vi "0 Main Application - Energy Usage Version B.vi"() -> ()   [LabVIEW 2018]
panel:
  out "selected file path":path
  out "Min Cluster":T1 {"Hour" format="%<%H:%M>t"}
  out "Max cluster":T2 {"Hour" format="%<%H:%M>t"}
  out "results  data file path":path
  in  "Print Button":bool
  out "Total usage per day (KWh)":dbl
  out "Total (kWh/day)":dbl[](array[numeric])
  in  "Just Week days":bool
  out "G-6:15PM-8:00PM":dbl format="%.1f"
  out "H-8:15PM-10:00PM":dbl format="%.1f"
  out "F-4:15PM-6:00PM":dbl format="%.1f"
  out "E-2:15PM-4:00PM":dbl format="%.1f"
  out "D-12:15 -2:00PM":dbl format="%.1f"
  out "C-10:15-12:00":dbl format="%.1f"
  out "B-8:15-10:00":dbl format="%.1f"
  out "A-6:15-8:00":dbl format="%.1f"
  out "Average usage":dbl[][](graph)
  out "standard deviation":dbl format="%0.2f"
  out "actual data":dbl[][](array[numeric])
  in  "Remove weekday fltr":bool
  in  "Weekday filter":T3
  in  "Remove filter":bool
  in  "Quarter Filter":T4 {"month ring" items=["Jan", "Feb", "Mar", "Apr", "May", "Jun", "Jul", "Ago", "Set", "Oct", "Nov", "Dec"]}
  in  "Tab Control":enum32{"per hour", "Total /day"}(tab)
  out "Per Hour":cluster{"Y":dbl[], "Y":dbl[]}[](graph)
  out "Average Demand (kW)":dbl format="%#.2g"
  out "Total Demand (KWh)":dbl format="%.2f"
  out "Total per day":cluster{"Y":dbl[], "Y":dbl[]}[](graph)
  out "Average Demand (KWh/day)":dbl
  in  "SAVE PEAK DATA":bool
  out "%":dbl[](array[numeric]) format="%.2f"
  out "Demand (KW)":dbl
  out "Profile per day":dbl[][](graph)
  out "Peaks":cluster{i32[], dbl[]}[](graph)
  out "Hour":i32 format="%<%H:%M>t"
  out "Energy Usage":dbl[][](graph)
  in  "Read file":bool
  in  "stop":bool
  out "Date":u16(ring) items=["Fri Jan 1 2010", "Sat Jan 2 2010", "Sun Jan 3 2010", "Mon Jan 4 2010", "Tue Jan 5 2010", "Wed Jan 6 2010", "Thu Jan 7 2010", "Fri Jan 8 2010", "Sat Jan 9 2010", "Sun Jan 10 2010", "Mon Jan 11 2010", "Tue Jan 12 2010", "Wed Jan 13 2010", "Thu Jan 14 2010", "Fri Jan 15 2010", "Sat Jan 16 2010", "Sun Jan 17 2010", "Mon Jan 18 2010", "Tue Jan 19 2010", "Wed Jan 20 2010", "Thu Jan 21 2010", "Fri Jan 22 2010", "Sat Jan 23 2010", "Sun Jan 24 2010", "Mon Jan 25 2010", "Tue Jan 26 2010", "Wed Jan 27 2010", "Thu Jan 28 2010", "Fri Jan 29 2010", "Sat Jan 30 2010", "Sun Jan 31 2010", "Mon Feb 1 2010", "Tue Feb 2 2010", "Wed Feb 3 2010", "Thu Feb 4 2010", "Fri Feb 5 2010", "Sat Feb 6 2010", "Sun Feb 7 2010", "Mon Feb 8 2010", "Tue Feb 9 2010", "Wed Feb 10 2010", "Thu Feb 11 2010", "Fri Feb 12 2010", "Sat Feb 13 2010", "Sun Feb 14 2010", "Mon Feb 15 2010", "Tue Feb 16 2010", "Wed Feb 17 2010", "Thu Feb 18 2010", "Fri Feb 19 2010", "Sat Feb 20 2010", "Sun Feb 21 2010", "Mon Feb 22 2010", "Tue Feb 23 2010", "Wed Feb 24 2010", "Thu Feb 25 2010", "Fri Feb 26 2010", "Sat Feb 27 2010", "Sun Feb 28 2010", "Mon Mar 1 2010", "Tue Mar 2 2010", "Wed Mar 3 2010", "Thu Mar 4 2010", "Fri Mar 5 2010", "Sat Mar 6 2010", "Sun Mar 7 2010", "Mon Mar 8 2010", "Tue Mar 9 2010", "Wed Mar 10 2010", "Thu Mar 11 2010", "Fri Mar 12 2010", "Sat Mar 13 2010", "Sun Mar 14 2010", "Mon Mar 15 2010", "Tue Mar 16 2010", "Wed Mar 17 2010", "Thu Mar 18 2010", "Fri Mar 19 2010", "Sat Mar 20 2010", "Sun Mar 21 2010", "Mon Mar 22 2010", "Tue Mar 23 2010", "Wed Mar 24 2010", "Thu Mar 25 2010", "Fri Mar 26 2010", "Sat Mar 27 2010", "Sun Mar 28 2010", "Mon Mar 29 2010", "Tue Mar 30 2010", "Wed Mar 31 2010", "Thu Apr 1 2010", "Fri Apr 2 2010", "Sat Apr 3 2010", "Sun Apr 4 2010", "Mon Apr 5 2010", "Tue Apr 6 2010", "Wed Apr 7 2010", "Thu Apr 8 2010", "Fri Apr 9 2010", "Sat Apr 10 2010", "Sun Apr 11 2010", "Mon Apr 12 2010", "Tue Apr 13 2010", "Wed Apr 14 2010", "Thu Apr 15 2010", "Fri Apr 16 2010", "Sat Apr 17 2010", "Sun Apr 18 2010", "Mon Apr 19 2010", "Tue Apr 20 2010", "Wed Apr 21 2010", "Thu Apr 22 2010", "Fri Apr 23 2010", "Sat Apr 24 2010", "Sun Apr 25 2010", "Mon Apr 26 2010", "Tue Apr 27 2010", "Wed Apr 28 2010", "Thu Apr 29 2010", "Fri Apr 30 2010", "Sat May 1 2010", "Sun May 2 2010", "Mon May 3 2010", "Tue May 4 2010", "Wed May 5 2010", "Thu May 6 2010", "Fri May 7 2010", "Sat May 8 2010", "Sun May 9 2010", "Mon May 10 2010", "Tue May 11 2010", "Wed May 12 2010", "Thu May 13 2010", "Fri May 14 2010", "Sat May 15 2010", "Sun May 16 2010", "Mon May 17 2010", "Tue May 18 2010", "Wed May 19 2010", "Thu May 20 2010", "Fri May 21 2010", "Sat May 22 2010", "Sun May 23 2010", "Mon May 24 2010", "Tue May 25 2010", "Wed May 26 2010", "Thu May 27 2010", "Fri May 28 2010", "Sat May 29 2010", "Sun May 30 2010", "Mon May 31 2010", "Tue Jun 1 2010", "Wed Jun 2 2010", "Thu Jun 3 2010", "Fri Jun 4 2010", "Sat Jun 5 2010", "Sun Jun 6 2010", "Mon Jun 7 2010", "Tue Jun 8 2010", "Wed Jun 9 2010", "Thu Jun 10 2010", "Fri Jun 11 2010", "Sat Jun 12 2010", "Sun Jun 13 2010", "Mon Jun 14 2010", "Tue Jun 15 2010", "Wed Jun 16 2010", "Thu Jun 17 2010", "Fri Jun 18 2010", "Sat Jun 19 2010", "Sun Jun 20 2010", "Mon Jun 21 2010", "Tue Jun 22 2010", "Wed Jun 23 2010", "Thu Jun 24 2010", "Fri Jun 25 2010", "Sat Jun 26 2010", "Sun Jun 27 2010", "Mon Jun 28 2010", "Tue Jun 29 2010", "Wed Jun 30 2010", "Thu Jul 1 2010", "Fri Jul 2 2010", "Sat Jul 3 2010", "Sun Jul 4 2010", "Mon Jul 5 2010", "Tue Jul 6 2010", "Wed Jul 7 2010", "Thu Jul 8 2010", "Fri Jul 9 2010", "Sat Jul 10 2010", "Sun Jul 11 2010", "Mon Jul 12 2010", "Tue Jul 13 2010", "Wed Jul 14 2010", "Thu Jul 15 2010", "Fri Jul 16 2010", "Sat Jul 17 2010", "Sun Jul 18 2010", "Mon Jul 19 2010", "Tue Jul 20 2010", "Wed Jul 21 2010", "Thu Jul 22 2010", "Fri Jul 23 2010", "Sat Jul 24 2010", "Sun Jul 25 2010", "Mon Jul 26 2010", "Tue Jul 27 2010", "Wed Jul 28 2010", "Thu Jul 29 2010", "Fri Jul 30 2010", "Sat Jul 31 2010", "Sun Aug 1 2010", "Mon Aug 2 2010", "Tue Aug 3 2010", "Wed Aug 4 2010", "Thu Aug 5 2010", "Fri Aug 6 2010", "Sat Aug 7 2010", "Sun Aug 8 2010", "Mon Aug 9 2010", "Tue Aug 10 2010", "Wed Aug 11 2010", "Thu Aug 12 2010", "Fri Aug 13 2010", "Sat Aug 14 2010", "Sun Aug 15 2010", "Mon Aug 16 2010", "Tue Aug 17 2010", "Wed Aug 18 2010", "Thu Aug 19 2010", "Fri Aug 20 2010", "Sat Aug 21 2010", "Sun Aug 22 2010", "Mon Aug 23 2010", "Tue Aug 24 2010", "Wed Aug 25 2010", "Thu Aug 26 2010", "Fri Aug 27 2010", "Sat Aug 28 2010", "Sun Aug 29 2010", "Mon Aug 30 2010", "Tue Aug 31 2010", "Wed Sep 1 2010", "Thu Sep 2 2010", "Fri Sep 3 2010", "Sat Sep 4 2010", "Sun Sep 5 2010", "Mon Sep 6 2010", "Tue Sep 7 2010", "Wed Sep 8 2010", "Thu Sep 9 2010", "Fri Sep 10 2010", "Sat Sep 11 2010", "Sun Sep 12 2010", "Mon Sep 13 2010", "Tue Sep 14 2010", "Wed Sep 15 2010", "Thu Sep 16 2010", "Fri Sep 17 2010", "Sat Sep 18 2010", "Sun Sep 19 2010", "Mon Sep 20 2010", "Tue Sep 21 2010", "Wed Sep 22 2010", "Thu Sep 23 2010", "Fri Sep 24 2010", "Sat Sep 25 2010", "Sun Sep 26 2010", "Mon Sep 27 2010", "Tue Sep 28 2010", "Wed Sep 29 2010", "Thu Sep 30 2010", "Fri Oct 1 2010", "Sat Oct 2 2010", "Sun Oct 3 2010", "Mon Oct 4 2010", "Tue Oct 5 2010", "Wed Oct 6 2010", "Thu Oct 7 2010", "Fri Oct 8 2010", "Sat Oct 9 2010", "Sun Oct 10 2010", "Mon Oct 11 2010", "Tue Oct 12 2010", "Wed Oct 13 2010", "Thu Oct 14 2010", "Fri Oct 15 2010", "Sat Oct 16 2010", "Sun Oct 17 2010", "Mon Oct 18 2010", "Tue Oct 19 2010", "Wed Oct 20 2010", "Thu Oct 21 2010", "Fri Oct 22 2010", "Sat Oct 23 2010", "Sun Oct 24 2010", "Mon Oct 25 2010", "Tue Oct 26 2010", "Wed Oct 27 2010", "Thu Oct 28 2010", "Fri Oct 29 2010", "Sat Oct 30 2010", "Sun Oct 31 2010", "Mon Nov 1 2010", "Tue Nov 2 2010", "Wed Nov 3 2010", "Thu Nov 4 2010", "Fri Nov 5 2010", "Sat Nov 6 2010", "Sun Nov 7 2010", "Mon Nov 8 2010", "Tue Nov 9 2010", "Wed Nov 10 2010", "Thu Nov 11 2010", "Fri Nov 12 2010", "Sat Nov 13 2010", "Sun Nov 14 2010", "Mon Nov 15 2010", "Tue Nov 16 2010", "Wed Nov 17 2010", "Thu Nov 18 2010", "Fri Nov 19 2010", "Sat Nov 20 2010", "Sun Nov 21 2010", "Mon Nov 22 2010", "Tue Nov 23 2010", "Wed Nov 24 2010", "Thu Nov 25 2010", "Fri Nov 26 2010", "Sat Nov 27 2010", "Sun Nov 28 2010", "Mon Nov 29 2010", "Tue Nov 30 2010", "Wed Dec 1 2010", "Thu Dec 2 2010", "Fri Dec 3 2010", "Sat Dec 4 2010", "Sun Dec 5 2010", "Mon Dec 6 2010", "Tue Dec 7 2010", "Wed Dec 8 2010", "Thu Dec 9 2010", "Fri Dec 10 2010", "Sat Dec 11 2010", "Sun Dec 12 2010", "Mon Dec 13 2010", "Tue Dec 14 2010", "Wed Dec 15 2010", "Thu Dec 16 2010", "Fri Dec 17 2010", "Sat Dec 18 2010", "Sun Dec 19 2010", "Mon Dec 20 2010", "Tue Dec 21 2010", "Wed Dec 22 2010", "Thu Dec 23 2010", "Fri Dec 24 2010", "Sat Dec 25 2010", "Sun Dec 26 2010", "Mon Dec 27 2010", "Tue Dec 28 2010", "Wed Dec 29 2010", "Thu Dec 30 2010", "Fri Dec 31 2010"]
  out "Peaks":dbl[](graph)
  # "A"
  # "B"
  # "C"
  # "D"
  # "E"
  # "F"
  # "G"
  # "H"
  # "```"
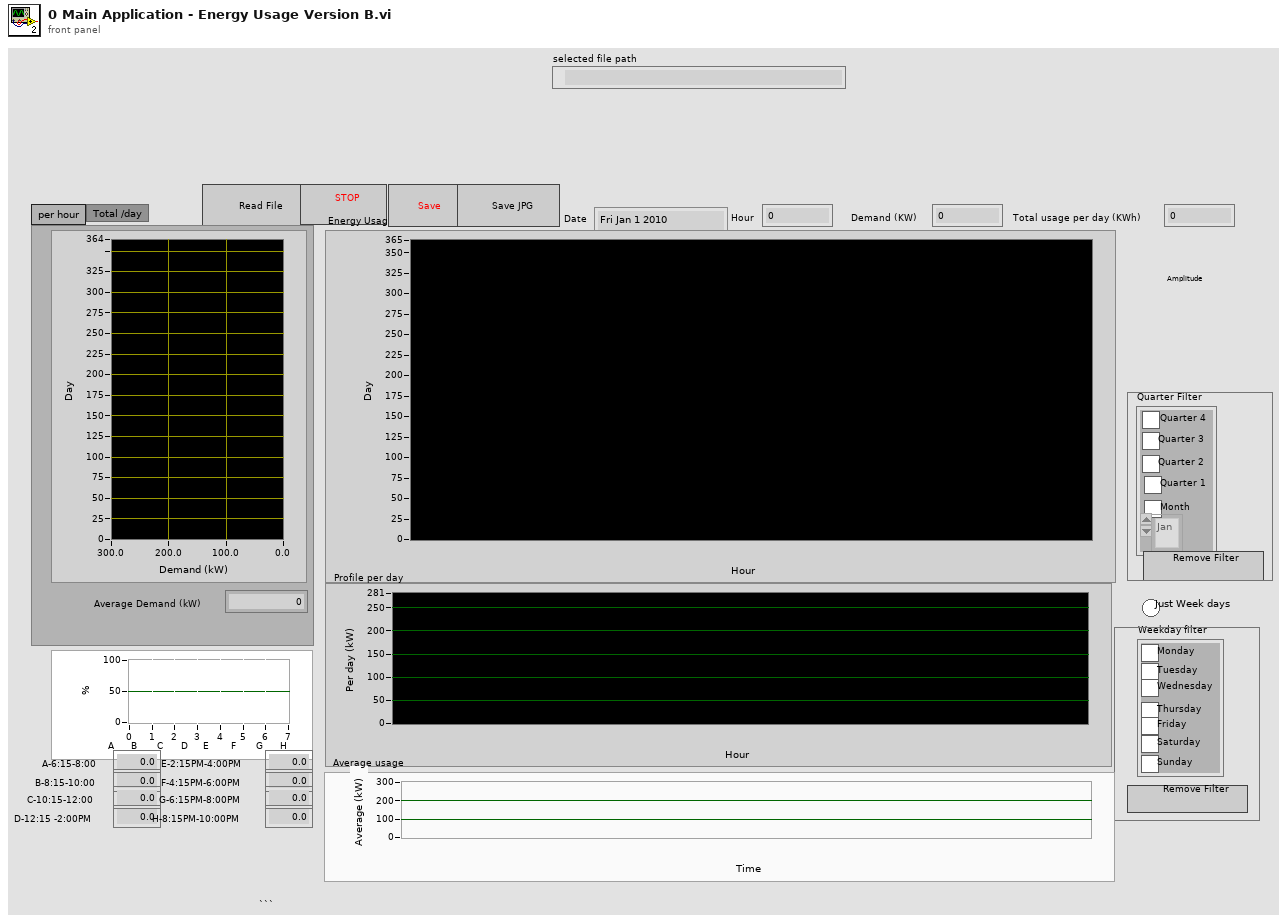
[diagram p1: front panel]
types:
  T1 = cluster{"Hour":i32, "min":dbl, "day of min":string}
  T2 = cluster{"Hour":i32, "Max peak":dbl, "day of max":string}
  T3 = cluster{"Monday":bool, "Tuesday":bool, "Wednesday":bool, "Thursday":bool, "Friday":bool, "Saturday":bool, "Sunday":bool}
  T4 = cluster{"Q1 3":bool, "Q2 2":bool, "Q3 2":bool, "Q4 2":bool, "Q1 4":bool, "month ring":u16}
  T5 = enum8{"Enabled", "Disabled", "Disabled and Grayed Out"}
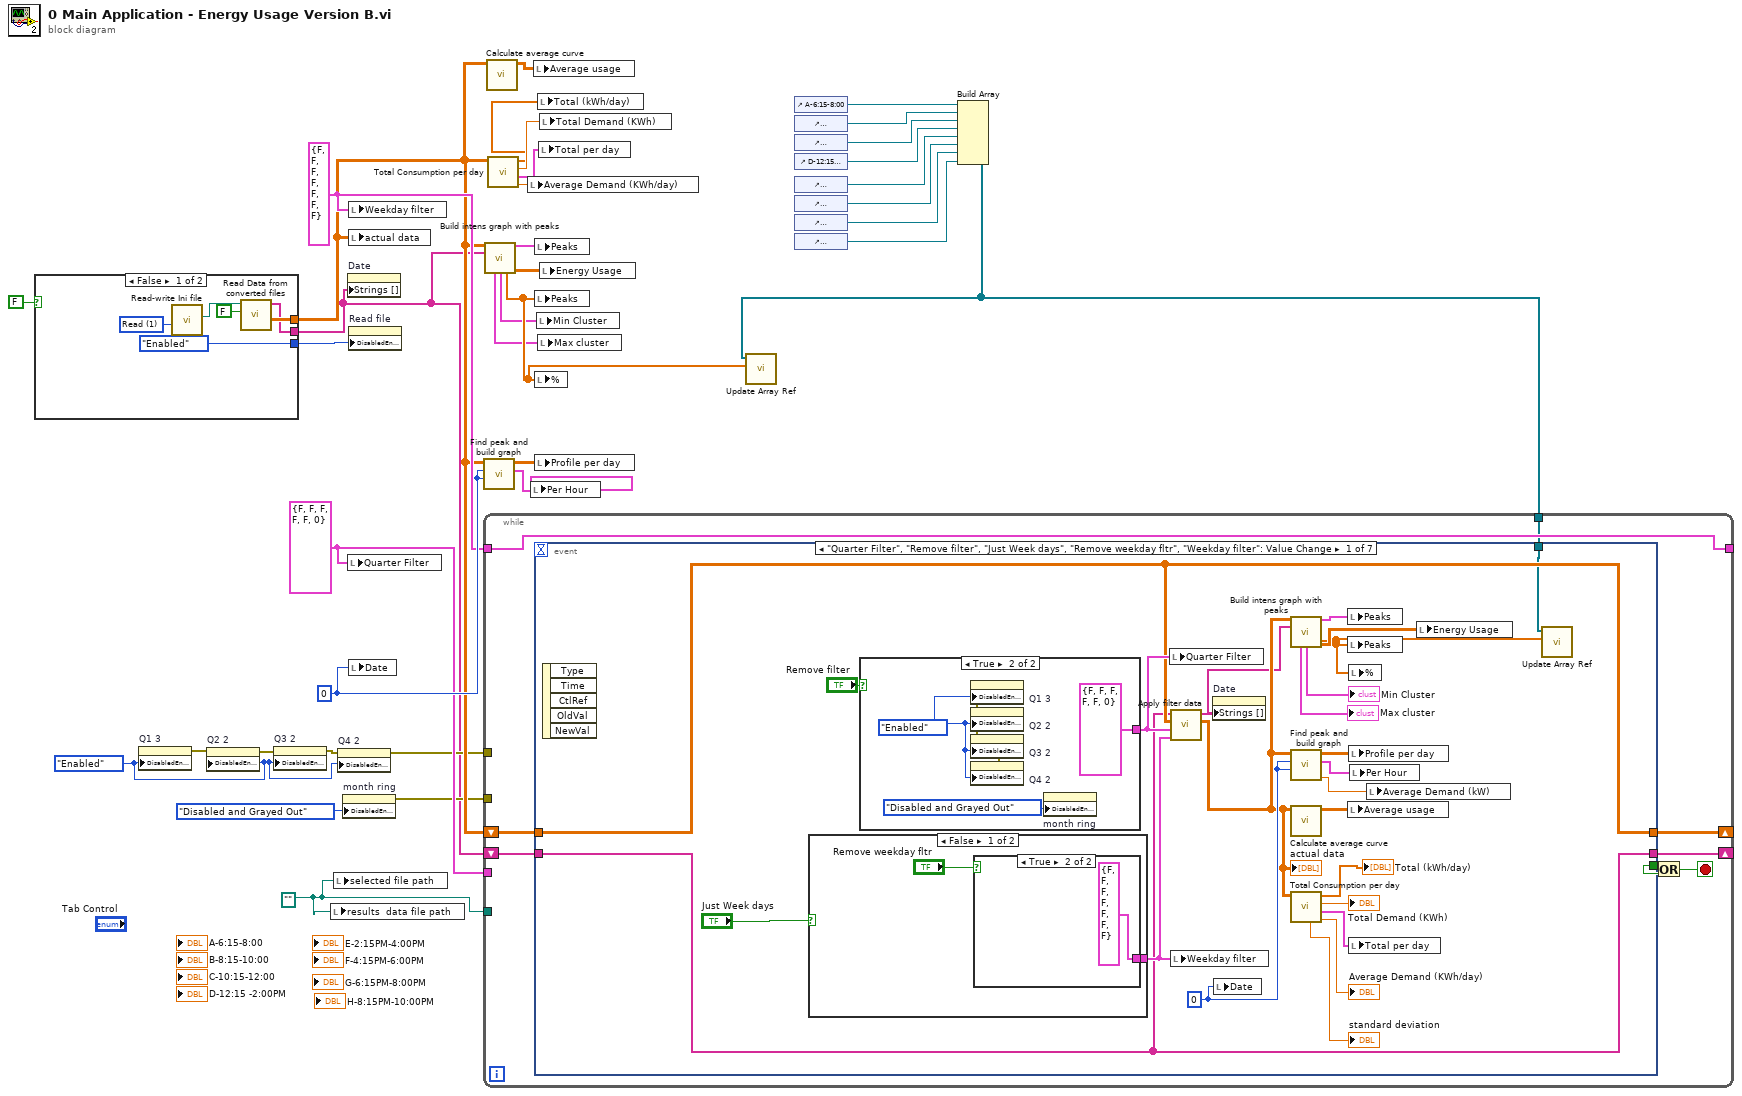
[diagram p0: block diagram]
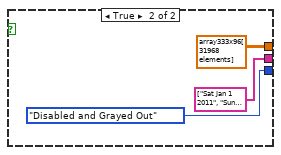
[diagram p2: hidden frame]
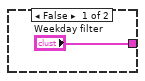
[diagram p3: hidden frame]
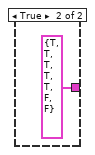
[diagram p4: hidden frame]
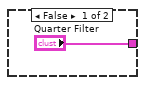
[diagram p5: hidden frame]
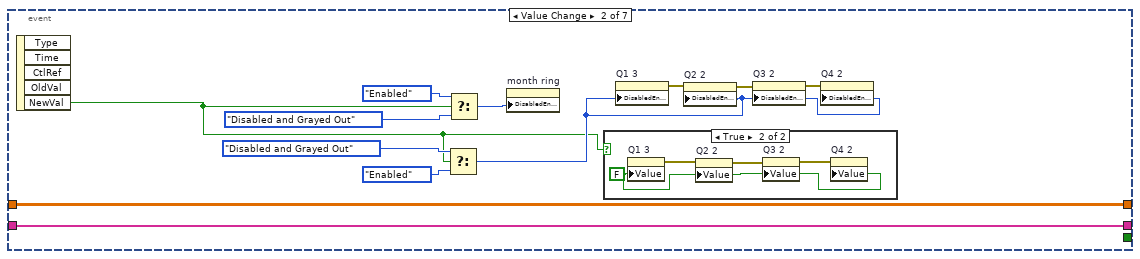
[diagram p6: hidden frame]
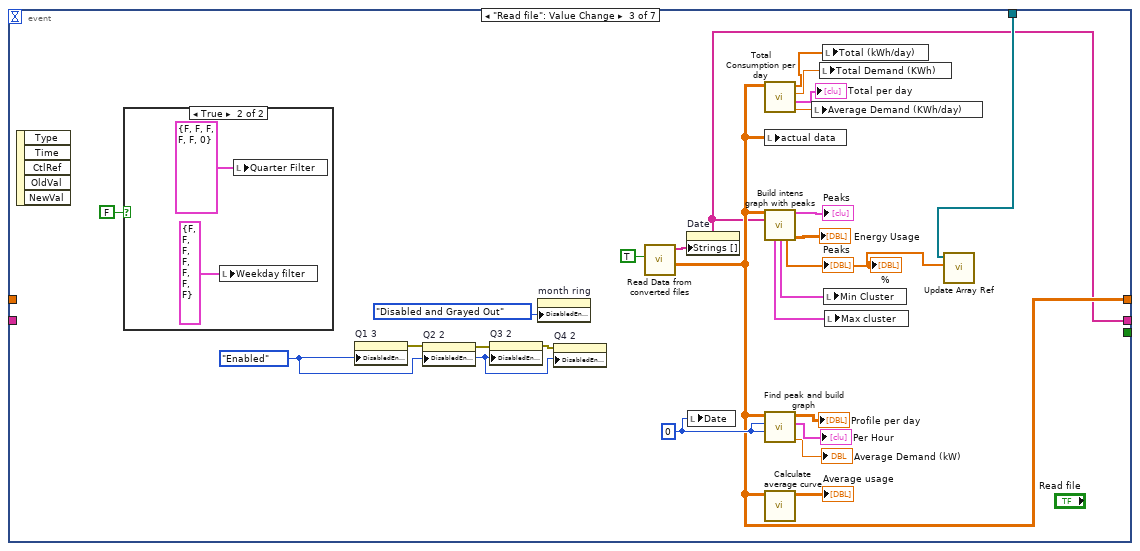
[diagram p8: hidden frame]
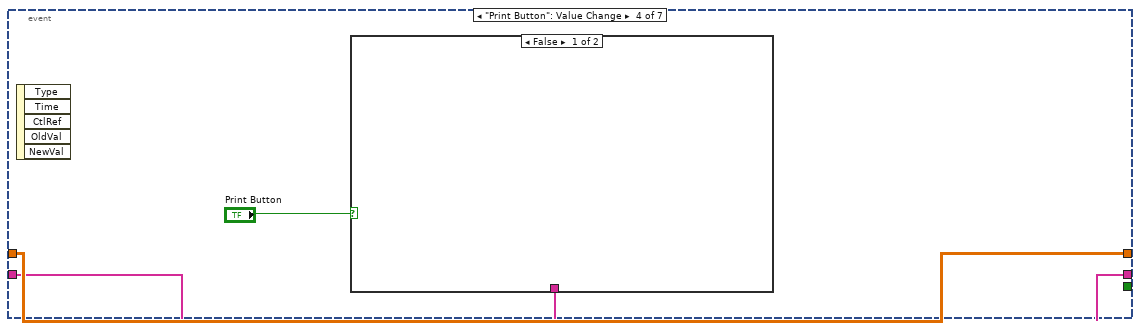
[diagram p10: hidden frame]
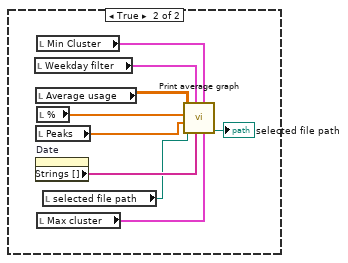
[diagram p11: hidden frame]
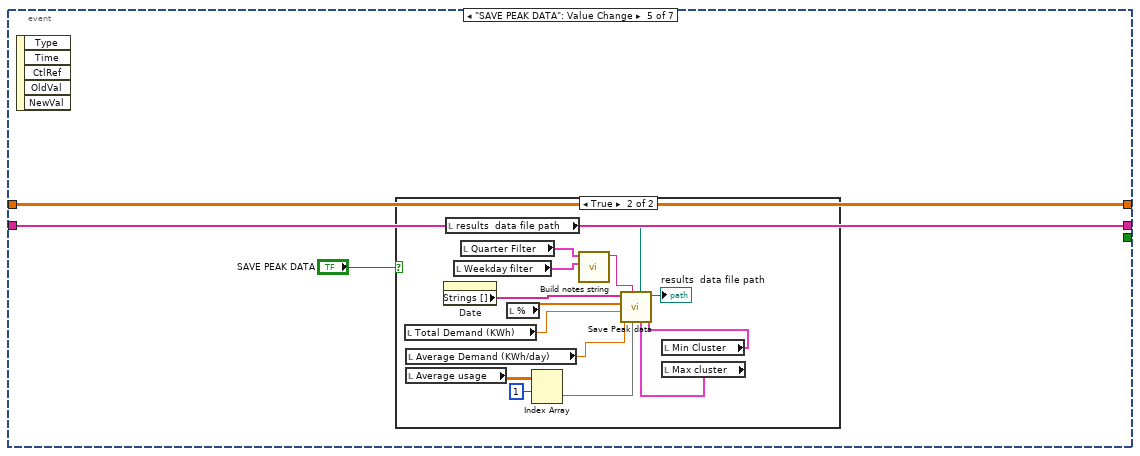
[diagram p12: hidden frame]
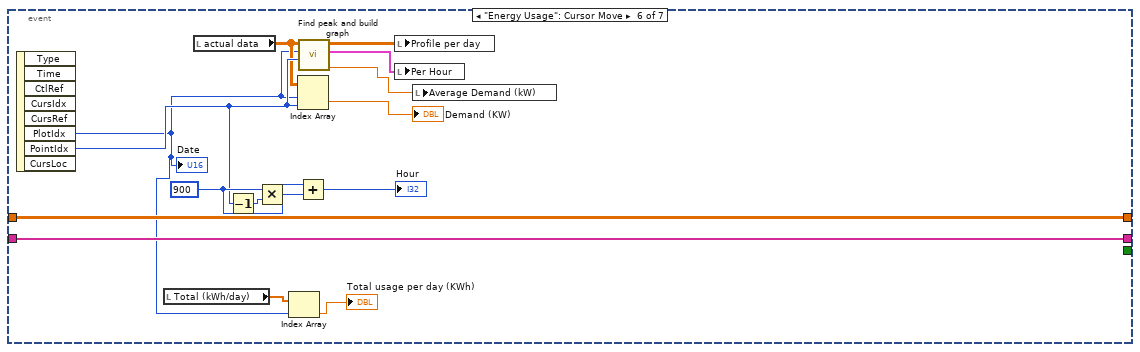
[diagram p14: hidden frame]
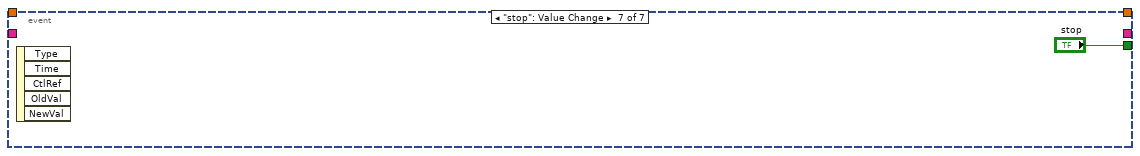
[diagram p15: hidden frame]
diagram:
  w1 = path ""
  w8 = T5."Enabled" ("Disabled")
  w31 = T4 {"Q1 3"=FALSE, "Q2 2"=FALSE, "Q3 2"=FALSE, "Q4 2"=FALSE, "Q1 4"=FALSE, "month ring"=0} ("Quarter Filter")
  w32 = T3 {"Monday"=FALSE, "Tuesday"=FALSE, "Wednesday"=FALSE, "Thursday"=FALSE, "Friday"=FALSE, "Saturday"=FALSE, "Sunday"=FALSE} ("Weekday filter")
  w33 = 0
  n1 = case shown="False" FALSE {
    tunnel: [w42 dbl[][] array333x96[31968 elements] ("actual data")] -> w25
    tunnel: [w41 string[] ["Sat Jan 1 2011", "Sun Jan 2 2011", "Mon Jan 3 2011", "Tue Jan 4 2011", "Wed Jan 5 2011", "Thu Jan 6 2011", "Fri Jan 7 2011", "Sat Jan 8 2011", "Sun Jan 9 2011", "Mon Jan 10 2011", "Tue Jan 11 2011", "Wed Jan 12 2011", "Thu Jan 13 2011", "Fri Jan 14 2011", "Sat Jan 15 2011", "Sun Jan 16 2011", "Mon Jan 17 2011", "Tue Jan 18 2011", "Wed Jan 19 2011", "Thu Jan 20 2011", "Fri Jan 21 2011", "Sat Jan 22 2011", "Sun Jan 23 2011", "Mon Jan 24 2011", "Tue Jan 25 2011", "Wed Jan 26 2011", "Thu Jan 27 2011", "Fri Jan 28 2011", "Sat Jan 29 2011", "Sun Jan 30 2011", "Mon Jan 31 2011", "Tue Feb 1 2011", "Wed Feb 2 2011", "Thu Feb 3 2011", "Fri Feb 4 2011", "Sat Feb 5 2011", "Sun Feb 6 2011", "Mon Feb 7 2011", "Tue Feb 8 2011", "Wed Feb 9 2011", "Thu Feb 10 2011", "Fri Feb 11 2011", "Sat Feb 12 2011", "Sun Feb 13 2011", "Mon Feb 14 2011", "Tue Feb 15 2011", "Wed Feb 16 2011", "Thu Feb 17 2011", "Fri Feb 18 2011", "Sat Feb 19 2011", "Sun Feb 20 2011", "Mon Feb 21 2011", "Tue Feb 22 2011", "Wed Feb 23 2011", "Thu Feb 24 2011", "Fri Feb 25 2011", "Sat Feb 26 2011", "Sun Feb 27 2011", "Mon Feb 28 2011", "Tue Mar 1 2011", "Wed Mar 2 2011", "Thu Mar 3 2011", "Fri Mar 4 2011", "Sat Mar 5 2011", "Sun Mar 6 2011", "Mon Mar 7 2011", "Tue Mar 8 2011", "Wed Mar 9 2011", "Thu Mar 10 2011", "Fri Mar 11 2011", "Sat Mar 12 2011", "Sun Mar 13 2011", "Mon Mar 14 2011", "Tue Mar 15 2011", "Wed Mar 16 2011", "Thu Mar 17 2011", "Fri Mar 18 2011", "Sat Mar 19 2011", "Sun Mar 20 2011", "Mon Mar 21 2011", "Tue Mar 22 2011", "Wed Mar 23 2011", "Thu Mar 24 2011", "Fri Mar 25 2011", "Sat Mar 26 2011", "Sun Mar 27 2011", "Mon Mar 28 2011", "Tue Mar 29 2011", "Wed Mar 30 2011", "Thu Mar 31 2011", "Fri Apr 1 2011", "Sat Apr 2 2011", "Sun Apr 3 2011", "Mon Apr 4 2011", "Tue Apr 5 2011", "Wed Apr 6 2011", "Thu Apr 7 2011", "Fri Apr 8 2011", "Sat Apr 9 2011", "Sun Apr 10 2011", "Mon Apr 11 2011", "Tue Apr 12 2011", "Wed Apr 13 2011", "Thu Apr 14 2011", "Fri Apr 15 2011", "Sat Apr 16 2011", "Sun Apr 17 2011", "Mon Apr 18 2011", "Tue Apr 19 2011", "Wed Apr 20 2011", "Thu Apr 21 2011", "Fri Apr 22 2011", "Sat Apr 23 2011", "Sun Apr 24 2011", "Mon Apr 25 2011", "Tue Apr 26 2011", "Wed Apr 27 2011", "Thu Apr 28 2011", "Fri Apr 29 2011", "Sat Apr 30 2011", "Sun May 1 2011", "Mon May 2 2011", "Tue May 3 2011", "Wed May 4 2011", "Thu May 5 2011", "Fri May 6 2011", "Sat May 7 2011", "Sun May 8 2011", "Mon May 9 2011", "Tue May 10 2011", "Wed May 11 2011", "Thu May 12 2011", "Fri May 13 2011", "Sat May 14 2011", "Sun May 15 2011", "Mon May 16 2011", "Tue May 17 2011", "Wed May 18 2011", "Thu May 19 2011", "Fri May 20 2011", "Sat May 21 2011", "Sun May 22 2011", "Mon May 23 2011", "Tue May 24 2011", "Wed May 25 2011", "Thu May 26 2011", "Fri May 27 2011", "Sat May 28 2011", "Sun May 29 2011", "Mon May 30 2011", "Tue May 31 2011", "Wed Jun 1 2011", "Thu Jun 2 2011", "Fri Jun 3 2011", "Sat Jun 4 2011", "Sun Jun 5 2011", "Mon Jun 6 2011", "Tue Jun 7 2011", "Wed Jun 8 2011", "Thu Jun 9 2011", "Fri Jun 10 2011", "Sat Jun 11 2011", "Sun Jun 12 2011", "Mon Jun 13 2011", "Tue Jun 14 2011", "Wed Jun 15 2011", "Thu Jun 16 2011", "Fri Jun 17 2011", "Sat Jun 18 2011", "Sun Jun 19 2011", "Mon Jun 20 2011", "Tue Jun 21 2011", "Wed Jun 22 2011", "Thu Jun 23 2011", "Fri Jun 24 2011", "Sat Jun 25 2011", "Sun Jun 26 2011", "Mon Jun 27 2011", "Tue Jun 28 2011", "Wed Jun 29 2011", "Thu Jun 30 2011", "Fri Jul 1 2011", "Sat Jul 2 2011", "Sun Jul 3 2011", "Mon Jul 4 2011", "Tue Jul 5 2011", "Wed Jul 6 2011", "Thu Jul 7 2011", "Fri Jul 8 2011", "Sat Jul 9 2011", "Sun Jul 10 2011", "Mon Jul 11 2011", "Tue Jul 12 2011", "Wed Jul 13 2011", "Thu Jul 14 2011", "Fri Jul 15 2011", "Sat Jul 16 2011", "Sun Jul 17 2011", "Mon Jul 18 2011", "Tue Jul 19 2011", "Wed Jul 20 2011", "Thu Jul 21 2011", "Fri Jul 22 2011", "Sat Jul 23 2011", "Sun Jul 24 2011", "Mon Jul 25 2011", "Tue Jul 26 2011", "Wed Jul 27 2011", "Thu Jul 28 2011", "Fri Jul 29 2011", "Sat Jul 30 2011", "Sun Jul 31 2011", "Mon Aug 1 2011", "Tue Aug 2 2011", "Wed Aug 3 2011", "Thu Aug 4 2011", "Fri Aug 5 2011", "Sat Aug 6 2011", "Sun Aug 7 2011", "Mon Aug 8 2011", "Tue Aug 9 2011", "Wed Aug 10 2011", "Thu Aug 11 2011", "Fri Aug 12 2011", "Sat Aug 13 2011", "Sun Aug 14 2011", "Mon Aug 15 2011", "Tue Aug 16 2011", "Wed Aug 17 2011", "Thu Aug 18 2011", "Fri Aug 19 2011", "Sat Aug 20 2011", "Sun Aug 21 2011", "Mon Aug 22 2011", "Tue Aug 23 2011", "Wed Aug 24 2011", "Thu Aug 25 2011", "Fri Aug 26 2011", "Sat Aug 27 2011", "Sun Aug 28 2011", "Mon Aug 29 2011", "Tue Aug 30 2011", "Wed Aug 31 2011", "Thu Sep 1 2011", "Fri Sep 2 2011", "Sat Sep 3 2011", "Sun Sep 4 2011", "Mon Sep 5 2011", "Tue Sep 6 2011", "Wed Sep 7 2011", "Thu Sep 8 2011", "Fri Sep 9 2011", "Sat Sep 10 2011", "Sun Sep 11 2011", "Mon Sep 12 2011", "Tue Sep 13 2011", "Wed Sep 14 2011", "Thu Sep 15 2011", "Fri Sep 16 2011", "Sat Sep 17 2011", "Sun Sep 18 2011", "Mon Sep 19 2011", "Tue Sep 20 2011", "Wed Sep 21 2011", "Thu Sep 22 2011", "Fri Sep 23 2011", "Sat Sep 24 2011", "Sun Sep 25 2011", "Mon Sep 26 2011", "Tue Sep 27 2011", "Wed Sep 28 2011", "Thu Sep 29 2011", "Fri Sep 30 2011", "Sat Oct 1 2011", "Sun Oct 2 2011", "Mon Oct 3 2011", "Tue Oct 4 2011", "Wed Oct 5 2011", "Thu Oct 6 2011", "Fri Oct 7 2011", "Sat Oct 8 2011", "Sun Oct 9 2011", "Mon Oct 10 2011", "Tue Oct 11 2011", "Wed Oct 12 2011", "Thu Oct 13 2011", "Fri Oct 14 2011", "Sat Oct 15 2011", "Sun Oct 16 2011", "Mon Oct 17 2011", "Tue Oct 18 2011", "Wed Oct 19 2011", "Thu Oct 20 2011", "Fri Oct 21 2011", "Sat Oct 22 2011", "Sun Oct 23 2011", "Mon Oct 24 2011", "Tue Oct 25 2011", "Wed Oct 26 2011", "Thu Oct 27 2011", "Fri Oct 28 2011", "Sat Oct 29 2011", "Sun Oct 30 2011", "Mon Oct 31 2011", "Tue Nov 1 2011", "Wed Nov 2 2011", "Thu Nov 3 2011", "Fri Nov 4 2011", "Sat Nov 5 2011", "Sun Nov 6 2011", "Mon Nov 7 2011", "Tue Nov 8 2011", "Wed Nov 9 2011", "Thu Nov 10 2011", "Fri Nov 11 2011", "Sat Nov 12 2011", "Sun Nov 13 2011", "Mon Nov 14 2011", "Tue Nov 15 2011", "Wed Nov 16 2011", "Thu Nov 17 2011", "Fri Nov 18 2011", "Sat Nov 19 2011", "Sun Nov 20 2011", "Mon Nov 21 2011", "Tue Nov 22 2011", "Wed Nov 23 2011", "Thu Nov 24 2011", "Fri Nov 25 2011", "Sat Nov 26 2011", "Sun Nov 27 2011", "Mon Nov 28 2011", "Tue Nov 29 2011"] ("dates")] -> w4
    tunnel: [T5."Enabled" ("Disabled") T5."Disabled and Grayed Out" ("Disabled")] -> w28
    frame False {
      w38 = u16 1 items=["Write", "Read"] ("OPERATION")
      n2 = call "Read-write Ini file.vi"("OPERATION"=w38) -> ("LAST DATA FILE 2"=w39:path)  [unwired: 10 in]
      n3 = call "Read Data from converted files.vi"("Open Dialog"=FALSE, "File Control"=w39) -> ("data"=w42:dbl[][], "dates"=w41:string[])  [unwired: 7 in, 1 out]
    }
    frame True {
    }
  }
  n4 = property on="Q1 3" class="Bool (strict)"("DisabledEnum"=w8) -> (error out=w11:errorcluster)  [unwired: 2 in, 1 out]
  n5 = property on="Q2 2" class="Bool (strict)"(error in=w11, "DisabledEnum"=w8) -> (error out=w9:errorcluster)  [unwired: 1 in, 1 out]
  n6 = property on="Q3 2" class="Bool (strict)"(error in=w9, "DisabledEnum"=w8) -> (error out=w10:errorcluster)  [unwired: 1 in, 1 out]
  n7 = local write "results  data file path"(w1) -> ()
  n8 = local write "selected file path"(w1) -> ()
  n9 = property on="Q4 2" class="Bool (strict)"(error in=w10, "DisabledEnum"=w8) -> (error out=w7:errorcluster)  [unwired: 1 in, 1 out]
  n10 = property on="month ring" class="Ring (strict)"("DisabledEnum"=T5."Disabled and Grayed Out" ("Disabled")) -> (error out=w22:errorcluster)  [unwired: 2 in, 1 out]
  n11 = property on="Date" class="Ring (strict)"("Strings []"=w4) -> ()  [unwired: 2 in, 2 out]
  n12 = local write "Quarter Filter"(w31) -> ()
  n13 = local write "Weekday filter"(w32) -> ()
  n14 = local write "actual data"(w25) -> ()
  n15 = property on="Read file" class="Bool"("DisabledEnum"=w28) -> ()  [unwired: 2 in, 2 out]
  n16 = local write "Date"(w33) -> ()
  n17 = call "Find peak and build graph.vi"("hour"=w33, "date"=w33, "data"=w25) -> ("XY Graph"=w21:cluster{"Y":dbl[], "Y":dbl[]}[], "Profile per day"=w36:dbl[][])  [unwired: 2 in, 5 out]
  n18 = call "Build intens graph with peaks.vi"("data"=w25, "dates"=w4) -> ("Peaks"=w35:cluster{i32[], dbl[]}[], "Max cluster"=w2:T2, "Min Cluster"=w3:T1, "%"=w5:dbl[], "Intensity Graph"=w34:dbl[][])  [unwired: 8 in, 1 out]
  n19 = call "Calculate average curve.vi"("data"=w25) -> ("data 2"=w24:dbl[][])  [unwired: 9 in, 1 out]
  n20 = call "Total Consumption per day.vi"("data"=w25) -> ("mean"=w26:dbl, "XY Graph"=w30:cluster{"Y":dbl[], "Y":dbl[]}[], "total demand"=w27:dbl, "Total (kWh/day)"=w6:dbl[])  [unwired: 5 in, 2 out]
  n21 = local write "Average Demand (KWh/day)"(w26) -> ()
  n22 = local write "Per Hour"(w21) -> ()
  n23 = local write "Average usage"(w24) -> ()
  n24 = local write "Peaks"(w35) -> ()
  n25 = local write "Peaks"(w5) -> ()
  n26 = local write "%"(w5) -> ()
  n27 = local write "Profile per day"(w36) -> ()
  n28 = local write "Min Cluster"(w3) -> ()
  n29 = local write "Total (kWh/day)"(w6) -> ()
  n30 = local write "Max cluster"(w2) -> ()
  n31 = local write "Total per day"(w30) -> ()
  n32 = local write "Total Demand (KWh)"(w27) -> ()
  n33 = local write "Energy Usage"(w34) -> ()
  n34 = control-ref of="A-6:15-8:00"() -> (w20:refnum<vi>)
  n35 = control-ref of="B-8:15-10:00"() -> (w19:refnum<vi>)
  n36 = control-ref of="C-10:15-12:00"() -> (w18:refnum<vi>)
  n37 = control-ref of="D-12:15 -2:00PM"() -> (w17:refnum<vi>)
  n38 = control-ref of="E-2:15PM-4:00PM"() -> (w16:refnum<vi>)
  n39 = control-ref of="F-4:15PM-6:00PM"() -> (w15:refnum<vi>)
  n40 = control-ref of="G-6:15PM-8:00PM"() -> (w14:refnum<vi>)
  n41 = control-ref of="H-8:15PM-10:00PM"() -> (w13:refnum<vi>)
  n42 = Build Array(w20, w19, w18, w17, w16, w15, w14, w13) -> (w12:refnum<vi>[])
  n43 = while {
    shift-right: [w52] -> _
    shift-left: w25 -> [w53]
    shift-right: [w50] -> _
    shift-left: w4 -> [w51]
    tunnel: [w47] -> _
    tunnel: w32 -> [w47]
    tunnel: w31 -> [_]
    tunnel: w22 -> [_]
    tunnel: w12 -> [w46]
    tunnel: w7 -> [_]
    tunnel: w1 -> [_]
    stop <- w49 stop-if-true
    n44 = event shown="[0] \"Quarter Filter\", \"Remove filter\", \"Just Week days\", \"Remove weekday fltr\", \"Weekday filter\": Value Change" {
      selector: _ -> [_ _ _ _ _ _ _]
      dyn-events: _ -> [_ _ _ _ _ _ _]
      timeout: _ -> [_ _ _ _ _ _ _]
      tunnel: [_ _ _ _ _ _ "stop"] -> w48
      tunnel: w53 -> [w69 w97 _ w133 w145 w169 _]
      tunnel: [w69 w97 w120 w133 w145 w169 _] -> w52
      tunnel: w51 -> [w57 w98 _ w132 w144 w168 _]
      tunnel: [w57 w98 w106 w132 w144 w168 _] -> w50
      tunnel: w46 -> [w62 _ w119 _ _ _ _]
      event "Quarter Filter", "Remove filter", "Just Week days", "Remove weekday fltr", "Weekday filter": Value Change {
        w68 = 0
        n45 = event-data() -> ()  [unwired: 1 in, 5 out]
        n46 = case shown="False" "Just Week days" {
          tunnel: [w78 T3 {"Monday"=TRUE, "Tuesday"=TRUE, "Wednesday"=TRUE, "Thursday"=TRUE, "Friday"=TRUE, "Saturday"=FALSE, "Sunday"=FALSE} ("Weekday filter")] -> w75
          frame False {
            n47 = case shown="True" "Remove weekday fltr" {
              tunnel: ["Weekday filter" T3 {"Monday"=FALSE, "Tuesday"=FALSE, "Wednesday"=FALSE, "Thursday"=FALSE, "Friday"=FALSE, "Saturday"=FALSE, "Sunday"=FALSE} ("Weekday filter")] -> w78
              frame False {
              }
              frame True {
              }
            }
          }
          frame True {
          }
        }
        n48 = case shown="True" "Remove filter" {
          tunnel: ["Quarter Filter" T4 {"Q1 3"=FALSE, "Q2 2"=FALSE, "Q3 2"=FALSE, "Q4 2"=FALSE, "Q1 4"=FALSE, "month ring"=0} ("Quarter Filter")] -> w76
          frame False {
          }
          frame True {
            w87 = T5."Enabled" ("Disabled")
            n49 = property on="Q1 3" class="Bool (strict)"("DisabledEnum"=w87) -> (error out=w84:errorcluster)  [unwired: 2 in, 1 out]
            n50 = property on="Q2 2" class="Bool (strict)"(error in=w84, "DisabledEnum"=w87) -> (error out=w86:errorcluster)  [unwired: 1 in, 1 out]
            n51 = property on="Q3 2" class="Bool (strict)"(error in=w86, "DisabledEnum"=w87) -> (error out=w85:errorcluster)  [unwired: 1 in, 1 out]
            n52 = property on="Q4 2" class="Bool (strict)"(error in=w85, "DisabledEnum"=w87) -> ()  [unwired: 1 in, 2 out]
            n53 = property on="month ring" class="Ring (strict)"("DisabledEnum"=T5."Disabled and Grayed Out" ("Disabled")) -> ()  [unwired: 2 in, 2 out]
          }
        }
        n54 = local write "Quarter Filter"(w76) -> ()
        n55 = call "Apply filter data.vi"("Weekday filter"=w75, "Quarter Filter"=w76, "data"=w69, "dates in"=w57) -> ("data out"=w63:dbl[][], "dates out"=w54:string[])  [unwired: 6 in]
        "actual data" <- w63
        n56 = local write "Weekday filter"(w75) -> ()
        n57 = property on="Date" class="Ring (strict)"("Strings []"=w54) -> ()  [unwired: 2 in, 2 out]
        n58 = local write "Date"(w68) -> ()
        n59 = call "Build intens graph with peaks.vi"("data"=w63, "dates"=w54) -> ("Peaks"=w71:cluster{i32[], dbl[]}[], "Max cluster"=→"Max cluster":T2, "Min Cluster"=→"Min Cluster":T1, "%"=w58:dbl[], "Intensity Graph"=w74:dbl[][])  [unwired: 8 in, 1 out]
        n60 = call "Find peak and build graph.vi"("hour"=w68, "date"=w68, "data"=w63) -> ("Average usage /hour"=w61:dbl, "XY Graph"=w73:cluster{"Y":dbl[], "Y":dbl[]}[], "Profile per day"=w72:dbl[][])  [unwired: 2 in, 4 out]
        n61 = call "Calculate average curve.vi"("data"=w63) -> ("data 2"=w64:dbl[][])  [unwired: 9 in, 1 out]
        n62 = call "Total Consumption per day.vi"("data"=w63) -> ("mean"=→"Average Demand (KWh/day)":dbl, "XY Graph"=w70:cluster{"Y":dbl[], "Y":dbl[]}[], "total demand"=→"Total Demand (KWh)":dbl, "Total (kWh/day)"=→"Total (kWh/day)":dbl[], "standard deviation"=→"standard deviation":dbl)  [unwired: 5 in, 1 out]
        n63 = local write "Peaks"(w71) -> ()
        n64 = local write "Peaks"(w58) -> ()
        n65 = local write "Average usage"(w64) -> ()
        n66 = local write "%"(w58) -> ()
        n67 = local write "Profile per day"(w72) -> ()
        n68 = local write "Total per day"(w70) -> ()
        n69 = local write "Per Hour"(w73) -> ()
        n70 = local write "Average Demand (kW)"(w61) -> ()
        n71 = local write "Energy Usage"(w74) -> ()
        n72 = call "Update Array Ref.vi"("%"=w58, "appended array"=w62) -> ()  [unwired: 10 in]
      }
      event "Quarter Filter.Q1 4": Value Change {
        n73 = event-data() -> ("NewVal"=w90:bool)  [unwired: 1 in, 4 out]
        n74 = Select(t=T5."Disabled and Grayed Out" ("Disabled"), s=w90, f=T5."Enabled" ("Disabled")) -> (s? t:f=w91:T5)
        n75 = Select(t=T5."Enabled" ("Disabled"), s=w90, f=T5."Disabled and Grayed Out" ("Disabled")) -> (s? t:f=w99:T5)
        n76 = property on="month ring" class="Ring (strict)"("DisabledEnum"=w99) -> ()  [unwired: 2 in, 2 out]
        n77 = case shown="True" w90 {
          frame False {
          }
          frame True {
            w102 = FALSE ("Value")
            n78 = property on="Q1 3" class="Bool (strict)"("Value"=w102) -> (error out=w105:errorcluster)  [unwired: 2 in, 1 out]
            n79 = property on="Q2 2" class="Bool (strict)"(error in=w105, "Value"=w102) -> (error out=w103:errorcluster)  [unwired: 1 in, 1 out]
            n80 = property on="Q3 2" class="Bool (strict)"(error in=w103, "Value"=w102) -> (error out=w104:errorcluster)  [unwired: 1 in, 1 out]
            n81 = property on="Q4 2" class="Bool (strict)"(error in=w104, "Value"=w102) -> ()  [unwired: 1 in, 2 out]
          }
        }
        n82 = property on="Q1 3" class="Bool (strict)"("DisabledEnum"=w91) -> (error out=w94:errorcluster)  [unwired: 2 in, 1 out]
        n83 = property on="Q2 2" class="Bool (strict)"(error in=w94, "DisabledEnum"=w91) -> (error out=w96:errorcluster)  [unwired: 1 in, 1 out]
        n84 = property on="Q3 2" class="Bool (strict)"(error in=w96, "DisabledEnum"=w91) -> (error out=w95:errorcluster)  [unwired: 1 in, 1 out]
        n85 = property on="Q4 2" class="Bool (strict)"(error in=w95, "DisabledEnum"=w91) -> ()  [unwired: 1 in, 2 out]
      }
      event "Read file": Value Change {
        w114 = T5."Enabled" ("Disabled")
        w127 = 0
        n86 = event-data() -> ()  [unwired: 1 in, 5 out]
        n87 = case shown="True" FALSE {
          frame False {
          }
          frame True {
            n88 = local write "Weekday filter"(T3 {"Monday"=FALSE, "Tuesday"=FALSE, "Wednesday"=FALSE, "Thursday"=FALSE, "Friday"=FALSE, "Saturday"=FALSE, "Sunday"=FALSE} ("Weekday filter")) -> ()
            n89 = local write "Quarter Filter"(T4 {"Q1 3"=FALSE, "Q2 2"=FALSE, "Q3 2"=FALSE, "Q4 2"=FALSE, "Q1 4"=FALSE, "month ring"=0} ("Quarter Filter")) -> ()
          }
        }
        n90 = property on="Q1 3" class="Bool (strict)"("DisabledEnum"=w114) -> (error out=w115:errorcluster)  [unwired: 2 in, 1 out]
        n91 = property on="Q2 2" class="Bool (strict)"(error in=w115, "DisabledEnum"=w114) -> (error out=w117:errorcluster)  [unwired: 1 in, 1 out]
        n92 = property on="Q3 2" class="Bool (strict)"(error in=w117, "DisabledEnum"=w114) -> (error out=w116:errorcluster)  [unwired: 1 in, 1 out]
        n93 = property on="month ring" class="Ring (strict)"("DisabledEnum"=T5."Disabled and Grayed Out" ("Disabled")) -> ()  [unwired: 2 in, 2 out]
        n94 = property on="Q4 2" class="Bool (strict)"(error in=w116, "DisabledEnum"=w114) -> ()  [unwired: 1 in, 2 out]
        n95 = call "Read Data from converted files.vi"("Open Dialog"=TRUE) -> ("data"=w120:dbl[][], "dates"=w106:string[])  [unwired: 8 in, 1 out]
        n96 = property on="Date" class="Ring (strict)"("Strings []"=w106) -> ()  [unwired: 2 in, 2 out]
        n97 = local write "Date"(w127) -> ()
        n98 = call "Total Consumption per day.vi"("data"=w120) -> ("mean"=w123:dbl, "XY Graph"=→"Total per day":cluster{"Y":dbl[], "Y":dbl[]}[], "total demand"=w122:dbl, "Total (kWh/day)"=w111:dbl[])  [unwired: 5 in, 2 out]
        n99 = local write "actual data"(w120) -> ()
        n100 = call "Build intens graph with peaks.vi"("data"=w120, "dates"=w106) -> ("Peaks"=→"Peaks":cluster{i32[], dbl[]}[], "Max cluster"=w107:T2, "Min Cluster"=w108:T1, "%"=w109:dbl[], "Intensity Graph"=→"Energy Usage":dbl[][])  [unwired: 8 in, 1 out]
        "%" <- w109
        "Peaks" <- w109
        n101 = call "Find peak and build graph.vi"("hour"=w127, "date"=w127, "data"=w120) -> ("Average usage /hour"=→"Average Demand (kW)":dbl, "XY Graph"=→"Per Hour":cluster{"Y":dbl[], "Y":dbl[]}[], "Profile per day"=→"Profile per day":dbl[][])  [unwired: 2 in, 4 out]
        n102 = call "Calculate average curve.vi"("data"=w120) -> ("data 2"=→"Average usage":dbl[][])  [unwired: 9 in, 1 out]
        n103 = local write "Average Demand (KWh/day)"(w123) -> ()
        n104 = local write "Total Demand (KWh)"(w122) -> ()
        n105 = local write "Total (kWh/day)"(w111) -> ()
        n106 = local write "Min Cluster"(w108) -> ()
        n107 = local write "Max cluster"(w107) -> ()
        n108 = call "Update Array Ref.vi"("%"=w109, "appended array"=w119) -> ()  [unwired: 10 in]
      }
      event "Print Button": Value Change {
        n109 = event-data() -> ()  [unwired: 1 in, 5 out]
        n110 = case shown="False" "Print Button" {
          tunnel: w132 -> [_ _]
          frame False {
          }
          frame True {
            n111 = local read "Weekday filter"() -> (w140:T3)
            n112 = local read "Average usage"() -> (w143:dbl[][])
            n113 = local read "Peaks"() -> (w141:dbl[])
            n114 = property on="Date" class="Ring (strict)"() -> ("Strings []"=w139:string[])  [unwired: 2 in, 2 out]
            n115 = local read "Min Cluster"() -> (w137:T1)
            n116 = local read "%"() -> (w142:dbl[])
            n117 = local read "Max cluster"() -> (w138:T2)
            n118 = local read "selected file path"() -> (w135:path)
            n119 = call "Print average graph.vi"("Max cluster"=w138, "Min Cluster"=w137, "dates"=w139, "Weekday filter"=w140, "Input selected file path"=w135, "Peaks"=w141, "%"=w142, "data 2"=w143) -> ("selected file path"=→"selected file path":path)  [unwired: 3 in]
          }
        }
      }
      event "SAVE PEAK DATA": Value Change {
        n120 = event-data() -> ()  [unwired: 1 in, 5 out]
        n121 = case shown="True" "SAVE PEAK DATA" {
          frame False {
          }
          frame True {
            n122 = local read "Total Demand (KWh)"() -> (w158:dbl)
            n123 = local read "Average Demand (KWh/day)"() -> (w157:dbl)
            n124 = local read "Average usage"() -> (w156:dbl[][])
            n125 = property on="Date" class="Ring (strict)"() -> ("Strings []"=w160:string[])  [unwired: 2 in, 2 out]
            n126 = local read "results  data file path"() -> (w149:path)
            n127 = local read "Weekday filter"() -> (w152:T3)
            n128 = local read "Quarter Filter"() -> (w153:T4)
            n129 = local read "%"() -> (w159:dbl[])
            n130 = Index Array(array=w156, index (row)=1) -> (element=w154:dbl[])  [unwired: 1 in]
            n131 = call "Build notes string.vi"("Weekday filter"=w152, "Quarter Filter"=w153) -> ("spreadsheet string 2"=w151:string)  [unwired: 9 in]
            n132 = local read "Min Cluster"() -> (w148:T1)
            n133 = local read "Max cluster"() -> (w147:T2)
            n134 = call "Save Peak data.vi"("Min Cluster"=w148, "Max cluster"=w147, "file path (use dialog)"=w149, "Average profile"=w154, "Days"=w151, "Average Demand / day"=w157, "Total demand"=w158, "%"=w159, "Strings []"=w160) -> ("path"=→"results  data file path":path)  [unwired: 2 in]
          }
        }
      }
      event "Energy Usage": Cursor Move {
        w174 = 900
        n135 = event-data() -> ("PlotIdx"=w164:i32, "PointIdx"=w170:i32)  [unwired: 1 in, 6 out]
        "Date" <- w164
        n136 = local read "Total (kWh/day)"() -> (w165:dbl[])
        n137 = local read "actual data"() -> (w167:dbl[][])
        n138 = Decrement(x=w170) -> (x-1=w162:i32)
        n139 = Multiply(x=w174, y=w162) -> (x*y=w175:i32)
        n140 = Index Array(array=w165, index=w164) -> (element=→"Total usage per day (KWh)":dbl)
        n141 = Index Array(array=w167, index (row)=w164, index (col)=w170) -> (element=→"Demand (KW)":dbl)
        n142 = Add(x=w174, y=w175) -> (x+y=→"Hour":i32)
        n143 = call "Find peak and build graph.vi"("hour"=w170, "date"=w164, "data"=w167) -> ("Average usage /hour"=w166:dbl, "XY Graph"=w171:cluster{"Y":dbl[], "Y":dbl[]}[], "Profile per day"=w173:dbl[][])  [unwired: 2 in, 4 out]
        n144 = local write "Profile per day"(w173) -> ()
        n145 = local write "Per Hour"(w171) -> ()
        n146 = local write "Average Demand (kW)"(w166) -> ()
      }
      event "stop": Value Change {
        n147 = event-data() -> ()  [unwired: 1 in, 5 out]
      }
    }
    n148 = Or(x=w48, y=w48) -> (x .or. y?=w49:bool)
  }
  n149 = call "Update Array Ref.vi"("%"=w5, "appended array"=w12) -> ()  [unwired: 10 in]
